vi "headingChooser.vi"(10 "Waypoint Direction (relative to current heading)":i32(knob) scale=-180.0..180.0, 11 "Wind Direction (relative to current heading)":i32(knob) scale=-180.0..180.0) -> (3 "Best Angle":i32(knob) scale=-180.0..180.0)   [LabVIEW 2011]
panel:
  out "max goodness value":sgl
  out "Combined Goodness function":cluster{i32, i32, sgl[]}(graph)
  out "Goodness Functions":cluster{i32, i32, sgl[][]}(graph)
  # "1. Various inputs are collected"
  # "2. Using a 'goodness function', each input is \n    converted to a value between 0 and 1 at each angle."
  # "3. At each angle, the goodness values are multiplied \n    together to get an overall goodness value."
  # "4. The angle with the maximum overall \n    goodness value is chosen"
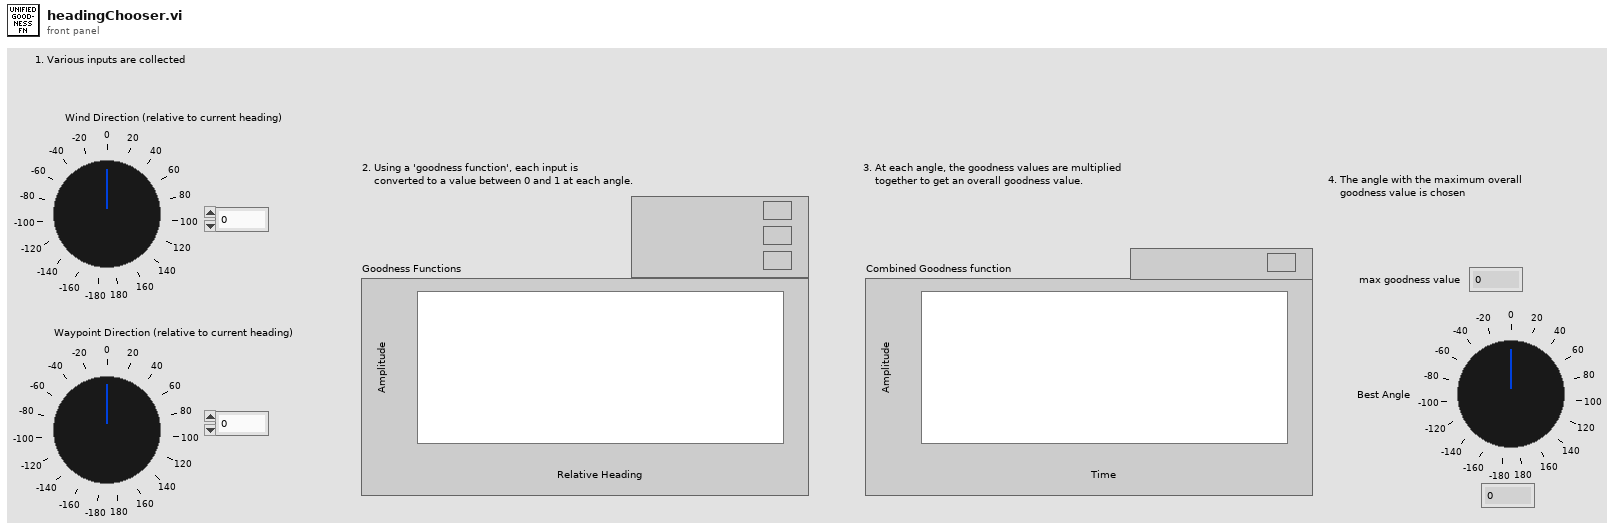
[diagram p1: front panel]
types:
  T1 = cluster{"min angle":i32, "resolution":i32, sgl[][]}
  T2 = cluster{"min angle":i32, "resolution":i32, sgl[]}
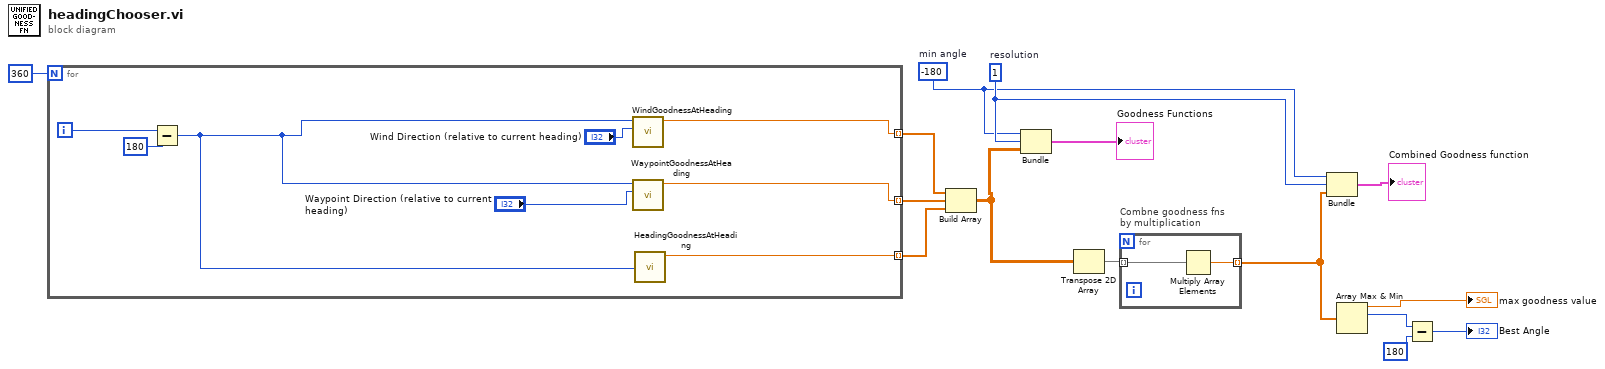
[diagram p0: block diagram]
diagram:
  w7 = 1  # resolution
  w6 = -180  # min angle
  n1 = for {
    N: 360 -> [_]
    tunnel: [w20] -> w13 mode=indexing
    tunnel: [w21] -> w12 mode=indexing
    tunnel: [w18] -> w1 mode=indexing
    i -> [w17]
    n2 = Subtract(x=w17, y=180) -> (x-y=w16:i32)
    n3 = call "WindGoodnessAtHeading.vi"("Wind Direction"="Wind Direction (relative to current heading)", "Heading"=w16) -> ("Wind goodness\nat this heading"=w20:sgl)  [unwired: 9 in]
    n4 = call "WaypointGoodnessAtHeading.vi"("Waypoint Direction"="Waypoint Direction (relative to current heading)", "Heading"=w16) -> ("Waypoint goodness\nat this heading"=w21:sgl)  [unwired: 9 in]
    n5 = call "HeadingGoodnessAtHeading.vi"("Heading"=w16) -> ("Heading goodness\nat this heading"=w18:sgl)  [unwired: 10 in]
  }
  n6 = Build Array(w13, w12, w1) -> (w11:sgl[][])
  n7 = Bundle("min angle"=w6, "resolution"=w7, w11) -> (→"Goodness Functions":T1)  [unwired: 1 in]
  n8 = Transpose 2D Array(2D array=w11) -> (transposed array=w10:sgl[][])
  n9 = for "Combne goodness fns\nby multiplication" {
    tunnel: w10 -> [w25] mode=indexing
    tunnel: [w24] -> w8 mode=indexing
    n10 = Multiply Array Elements(1:w25) -> (0:w24:sgl)
  }
  n11 = Bundle("min angle"=w6, "resolution"=w7, w8) -> (→"Combined Goodness function":T2)  [unwired: 1 in]
  n12 = Array Max & Min(array=w8) -> (max value=→"max goodness value":sgl, max index (indices)=w4:i32)  [unwired: 2 out]
  n13 = Subtract(x=w4, y=180) -> (x-y=→"Best Angle":i32)
